vi "Find Next Available DigPatrn FPGA Resource and Name.vi"(9 "FPGA Resources":string[](array[string]), 10 "Patterns":T1[](array[typedef]), 11 "New Pattern in":T1) -> (3 "New Pattern out":T1)   [LabVIEW 2017, in "Engine Simulation Toolkit System Explorer.lvlib"]
uses:
  Engine Simulation Toolkit System Explorer.lvlib
  Digital Pattern.ctl
  Digital Pattern Base.ctl
  Digital Pattern Remove Edge.ctl
  Digital Pattern Add Pulse.ctl
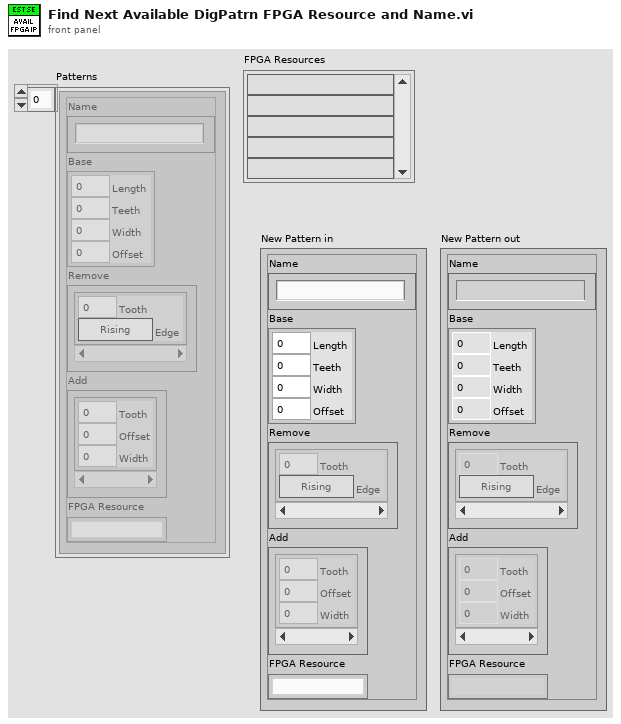
[diagram p1: front panel]
types:
  T1 = typedef "Engine Simulation Toolkit System Explorer.lvlib/Digital Pattern.ctl" = cluster{"Name":string, "Base":T2, "Remove":T3[], "Add":T4[], "FPGA Resource":string}
  T2 = typedef "Engine Simulation Toolkit System Explorer.lvlib/Digital Pattern Base.ctl" = cluster{"Length":dbl, "Teeth":u16, "Width":dbl, "Offset":dbl}
  T3 = typedef "Engine Simulation Toolkit System Explorer.lvlib/Digital Pattern Remove Edge.ctl" = cluster{"Tooth":u16, "Edge":bool}
  T4 = typedef "Engine Simulation Toolkit System Explorer.lvlib/Digital Pattern Add Pulse.ctl" = cluster{"Tooth":u16, "Offset":dbl, "Width":dbl}
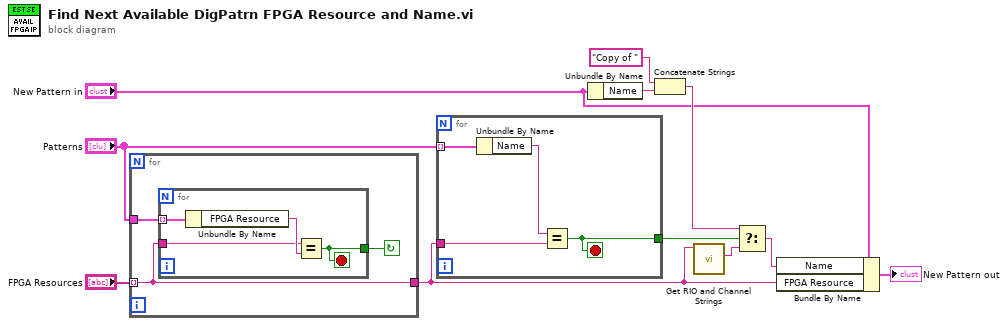
[diagram p0: block diagram]
diagram:
  n1 = for {
    tunnel: "FPGA Resources" -> [w13] mode=indexing
    tunnel: "Patterns" -> [w14]
    tunnel: [w13] -> w1
    stop <- w12 continue-if-true
    n2 = for {
      tunnel: w14 -> [w18] mode=indexing
      tunnel: w13 -> [w16]
      tunnel: [w15] -> w12
      stop <- w15 stop-if-true
      n3 = Unbundle By Name(w18) -> ("FPGA Resource"=w17:string)
      n4 = Equal?(x=w16, y=w17) -> (x = y?=w15:bool)
    }
  }
  n5 = for {
    tunnel: "Patterns" -> [w21] mode=indexing
    tunnel: w1 -> [w22]
    tunnel: [w19] -> w9
    stop <- w19 stop-if-true
    n6 = Unbundle By Name(w21) -> ("Name"=w20:string)
    n7 = Equal?(x=w20, y=w22) -> (x = y?=w19:bool)
  }
  n8 = Unbundle By Name("New Pattern in") -> ("Name"=w6:string)
  n9 = Concatenate Strings("Copy of " ("string"), w6) -> (w7:string)
  n10 = call "Get RIO and Channel Strings.vi"("rio/channel"=w1) -> ("channel"=w2:string)  [unwired: 9 in, 1 out]
  n11 = Select(t=w7, s=w9, f=w2) -> (s? t:f=w4:string)
  n12 = Bundle By Name(cluster="New Pattern in", "Name"=w4, "FPGA Resource"=w1) -> (→"New Pattern out":T1)
